vi "choreo_read_csv_FGV.vi"(9 "inTRAJECTORY":T1, 11 "Command":enum16{"Read Traj", "Write Traj"}(ring)) -> (1 "outTRAJECTORY":T1)   [LabVIEW 2019]
uses:
  <vilib>/Rock Robotics/WPI/ThirdParty/ChoreoLib/TypeDef/ChoreoTrajectoryState.ctl
  <vilib>/Rock Robotics/WPI/ThirdParty/ChoreoLib/ChoreoLib.lvlib
  <vilib>/Rock Robotics/WPI/ThirdParty/ChoreoLib/TypeDef/ChoreoTrajectory.ctl
panel:
  # "This is purposefully \n\nNOT re-entrant."
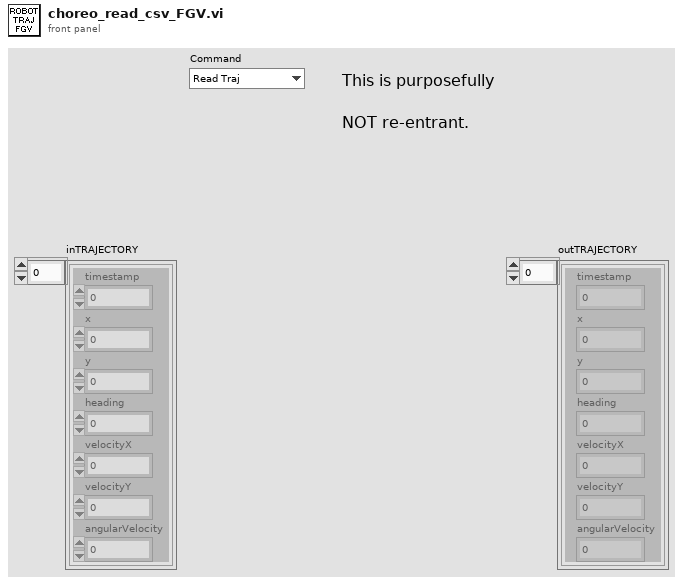
[diagram p1: front panel]
types:
  T1 = typedef "ChoreoLib.lvlib/ChoreoTrajectory.ctl" = T2[]
  T2 = typedef "ChoreoLib.lvlib/ChoreoTrajectoryState.ctl" = cluster{"timestamp":dbl, "x":dbl, "y":dbl, "heading":dbl, "velocityX":dbl, "velocityY":dbl, "angularVelocity":dbl}
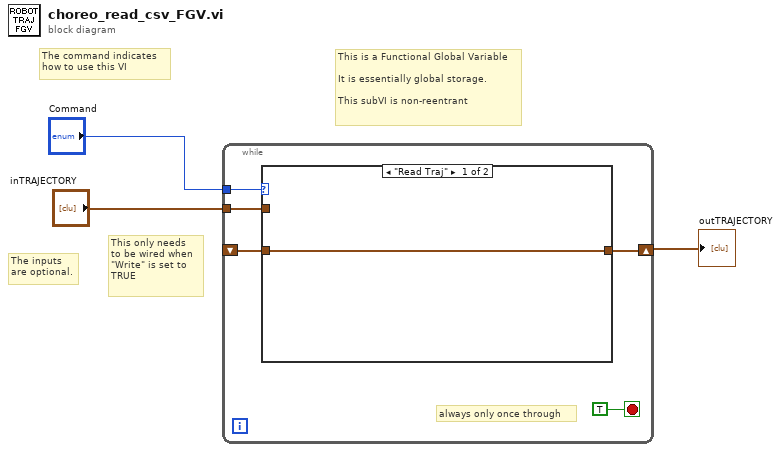
[diagram p0: block diagram]
diagram:
  # "This only needs\nto be wired when\n\"Write\" is set to\nTRUE"
  # "The command indicates\nhow to use this VI"
  # "The inputs \nare optional."
  # "This is a Functional Global Variable\n\nIt is essentially global storage.\n\nThis subVI is non-reentrant"
  n1 = while {
    tunnel: "Command" -> [w7]
    tunnel: "inTRAJECTORY" -> [w5]
    shift-right: [w6] -> w3
    shift-left: _ -> [w4]
    stop <- TRUE stop-if-true
    # "always only once through"
    n2 = case shown="\"Read Traj\"" w7 {
      tunnel: [w9 w10] -> w6
      tunnel: w5 -> [_ w10]
      tunnel: w4 -> [w9 _]
      frame "Read Traj" {
      }
      frame "Write Traj" {
        # "Save the trajectory\nin the shift \nregister."
      }
    }
  }
  "outTRAJECTORY" <- w3
